vi "Case Viewer.vi"(8 "Case":string, 10 "Flush?":bool, 11 "Str Refnum":refnum<vi>) -> (3 "Recent Cases":string)   [LabVIEW 2011]
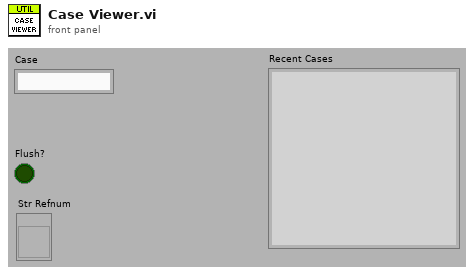
[diagram p1: front panel]
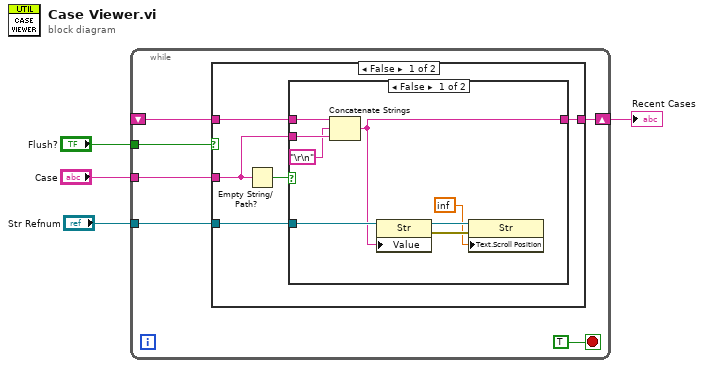
[diagram p0: block diagram]
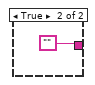
[diagram p3: hidden frame]
diagram:
  n1 = while {
    shift-right: [w9] -> w3
    shift-left: _ -> [w10]
    tunnel: "Case" -> [w8]
    tunnel: "Flush?" -> [w6]
    tunnel: "Str Refnum" -> [w5]
    stop <- TRUE stop-if-true
    n2 = case shown="False" w6 {
      tunnel: w10 -> [w15 _]
      tunnel: [w14 ""] -> w9
      tunnel: w8 -> [w13 _]
      tunnel: w5 -> [w11 _]
      frame False {
        n3 = Empty String/Path?(string/path=w13) -> (empty?=w12:bool)
        n4 = case shown="False" w12 {
          tunnel: w15 -> [w22 w24]
          tunnel: [w16 w24] -> w14
          tunnel: w13 -> [w23 _]
          tunnel: w11 -> [w21 _]
          frame False {
            n5 = Concatenate Strings(w22, "\r\n", w23) -> (w16:string)
            n6 = property class="Str"(reference=w21, "Value"=w16) -> (reference out=w19:refnum<vi>, error out=w18:errorcluster)  [unwired: 1 in]
            n7 = property class="Str"(reference=w19, error in=w18, "Text.Scroll Position"=inf) -> ()  [unwired: 2 out]
          }
          frame True {
          }
        }
      }
      frame True {
      }
    }
  }
  "Recent Cases" <- w3
